vi "select(sub).vi"(1 "element":refnum<vi>, 2 "appended array":refnum<vi>[](array[refnum]), 3 "Array":i32[](array[numeric])=[1, 2, 3, 4, 5, 1000, 1001, 1002, 1003, 0, 0]) -> (0 "element 2":i32)   [LabVIEW 2015]
panel:
  in  "stop 2":bool
  in  "Update value button":bool
  in  "Sweep freq. delay [ms]":dbl
  in  "Sweep freq. stop [Hz]":dbl format="%#_10p"
  in  "Sweep freq. incr [Hz]":dbl format="%#.10p"
  in  "Sweep freq. start [Hz]":dbl format="%#_10p"
  in  "Wave amplitude [mV]":dbl min=0.0 max=3000.0 step=1.0
  in  "Hardware Type":string(combo)="4"
  in  "Time Stamp":timestamp
  in  "Test waveform":string(combo)="1"
  in  "Current Frequency [Hz]":dbl min=0.0 step=1.0 format="%#.10p"
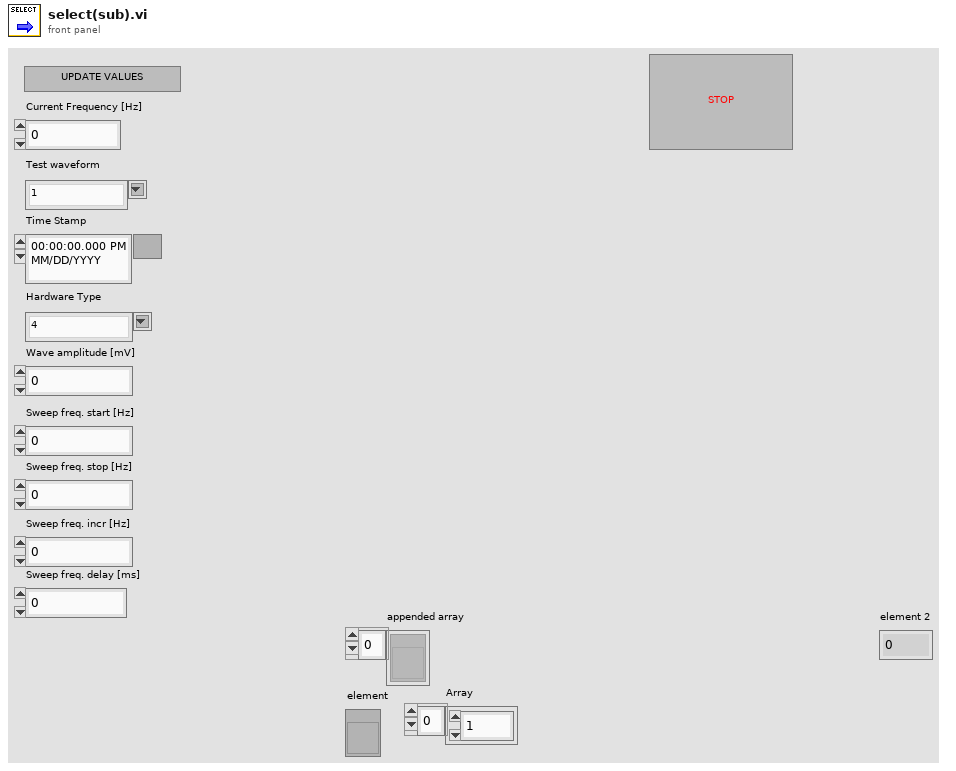
[diagram p1: front panel]
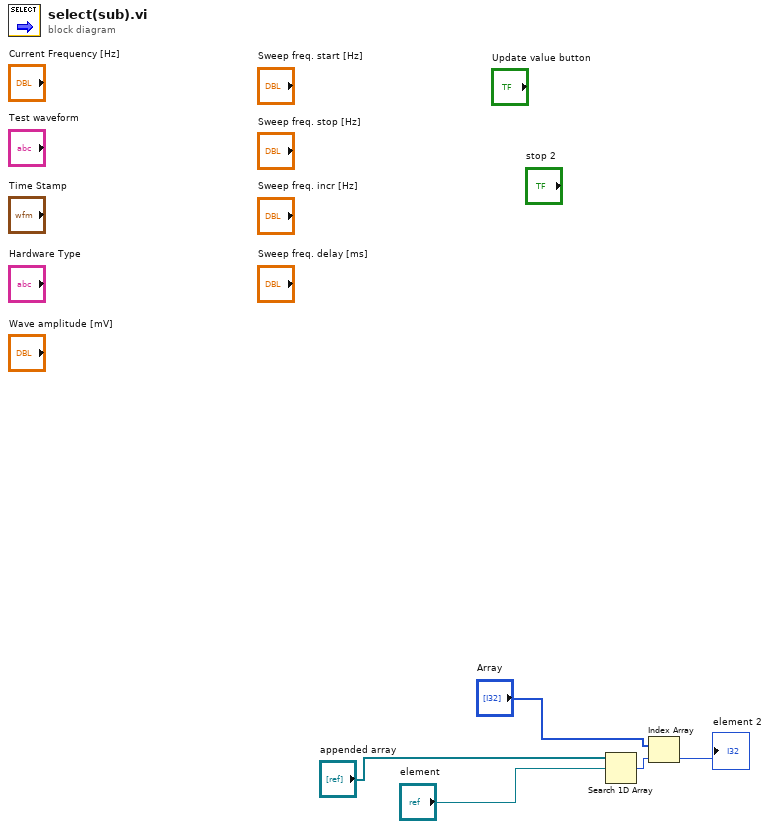
[diagram p0: block diagram]
diagram:
  n1 = Search 1D Array(1D array="appended array", element="element") -> (index of element=w5:i32)  [unwired: 1 in]
  n2 = Index Array(array="Array", index=w5) -> (element=→"element 2":i32)
